vi "Sort_2D Str.vi"(5 "정렬":enum16{"오름차순", "내림차순"}(ring), 7 "기준열":u16, 8 "error in (no error)":errorcluster caption="에러 입력(에러 없음)", 11 "Data in":string[][](array[string])) -> (0 "error out":errorcluster caption="에러 출력", 3 "Data out":string[][](array[string]))   [LabVIEW 2020]
panel:
  out "숫자?":bool
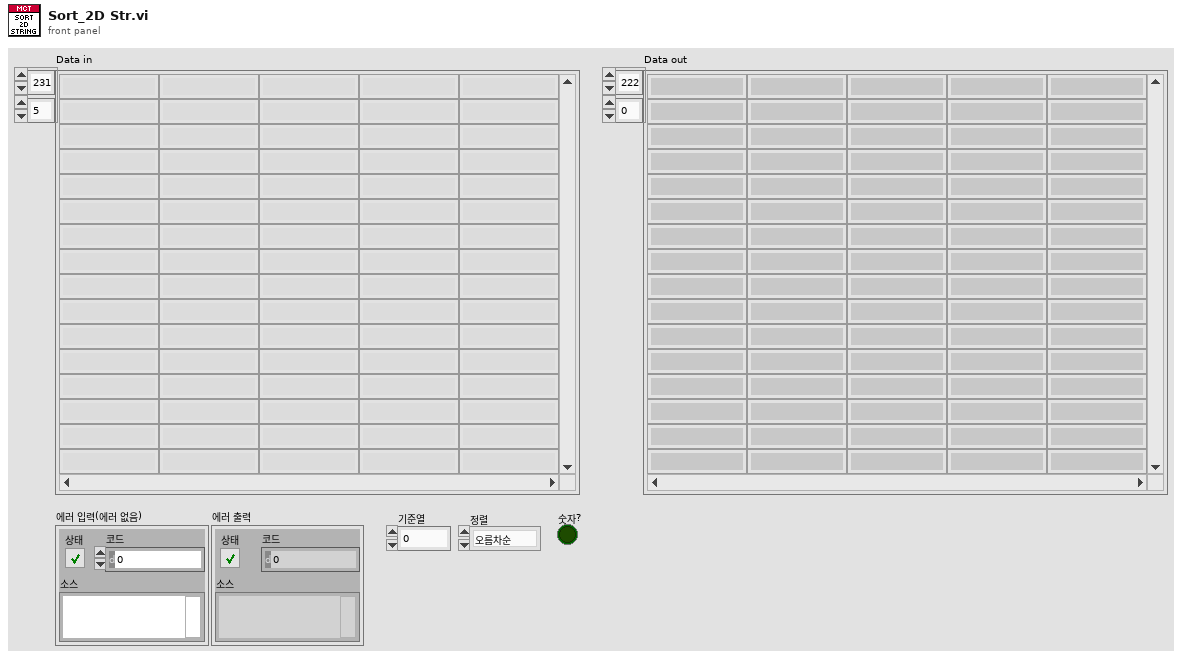
[diagram p1: front panel]
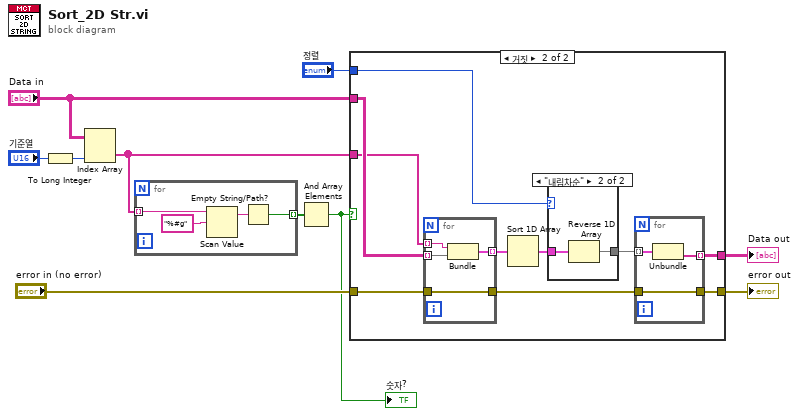
[diagram p0: block diagram]
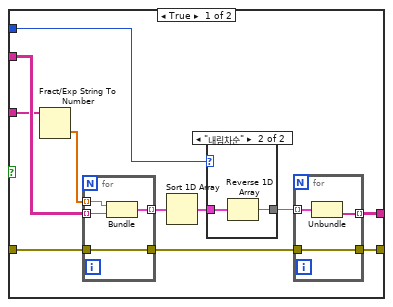
[diagram p2: hidden frame]
diagram:
  n1 = To Long Integer(number="기준열") -> (32bit integer=w9:i32)
  n2 = Index Array(array="Data in", index (col)=w9) -> (element=w3:string[])  [unwired: 1 in]
  n3 = for {
    tunnel: w3 -> [w14] mode=indexing
    tunnel: [w11] -> w2 mode=indexing
    n4 = Scan Value(string=w14, format string="%#g" ("포맷 문자열")) -> (output string=w12:string)  [unwired: 1 in, 1 out]
    n5 = Empty String/Path?(string/path=w12) -> (empty?=w11:bool)
  }
  n6 = And Array Elements(Boolean array=w2) -> (logical AND=w1:bool)
  "숫자?" <- w1
  n7 = case shown="거짓" w1 {
    tunnel: "Data in" -> [w25 w45]
    tunnel: [w24 w44] -> w7
    tunnel: [w23 w43] -> w6
    tunnel: "정렬" -> [w22 w42]
    tunnel: "error in (no error)" -> [w17 w37]
    tunnel: w3 -> [w16 w36]
    frame True {
      n8 = Fract/Exp String To Number(string=w16) -> (number=w15:dbl[])  [unwired: 3 in, 1 out]
      n9 = for {
        tunnel: w25 -> [w34] mode=indexing
        tunnel: w15 -> [w35] mode=indexing
        tunnel: [w33] -> w21 mode=indexing
        tunnel: w17 -> [w32]
        tunnel: [w32] -> w20
        n10 = Bundle("문자열"=w35, "Data in"=w34) -> (w33:cluster{"문자열":dbl, "Data in":string[]})  [unwired: 1 in]
      }
      n11 = Sort 1D Array(array=w21) -> (sorted array=w18:cluster{"문자열":dbl, "Data in":string[]}[])
      n12 = case shown="\"내림차순\"" w22 {
        tunnel: [w26 w27] -> w19
        tunnel: w18 -> [w26 w28]
        frame "오름차순", Default {
        }
        frame "내림차순" {
          n13 = Reverse 1D Array(array=w28) -> (reversed array=w27:cluster{"문자열":dbl, "Data in":string[]}[])
        }
      }
      n14 = for {
        tunnel: w19 -> [w31] mode=indexing
        tunnel: [w30] -> w24 mode=indexing
        tunnel: w20 -> [w29]
        tunnel: [w29] -> w23
        n15 = Unbundle(w31) -> ("Data in"=w30:string[])  [unwired: 1 out]
      }
    }
    frame False {
      n16 = for {
        tunnel: w45 -> [w54] mode=indexing
        tunnel: w36 -> [w55] mode=indexing
        tunnel: [w53] -> w41 mode=indexing
        tunnel: w37 -> [w52]
        tunnel: [w52] -> w40
        n17 = Bundle("문자열"=w55, "Data in"=w54) -> (w53:cluster{"문자열":string, "Data in":string[]})  [unwired: 1 in]
      }
      n18 = Sort 1D Array(array=w41) -> (sorted array=w38:cluster{"문자열":string, "Data in":string[]}[])
      n19 = case shown="\"내림차순\"" w42 {
        tunnel: [w46 w47] -> w39
        tunnel: w38 -> [w46 w48]
        frame "오름차순", Default {
        }
        frame "내림차순" {
          n20 = Reverse 1D Array(array=w48) -> (reversed array=w47:cluster{"문자열":string, "Data in":string[]}[])
        }
      }
      n21 = for {
        tunnel: w39 -> [w51] mode=indexing
        tunnel: [w50] -> w44 mode=indexing
        tunnel: w40 -> [w49]
        tunnel: [w49] -> w43
        n22 = Unbundle(w51) -> ("Data in"=w50:string[])  [unwired: 1 out]
      }
    }
  }
  "Data out" <- w7
  "error out" <- w6
